vi "Laurel Data GET Top Level.vi"(0 "Laurel IP Address":string="10.0.3.173", 1 "Laurel Serial Commands":T1, 2 "First Call?":bool, 5 "Use Delay":bool, 9 "Serial VISA":refnum<visa-resource-name>, 11 "error in (no error)":errorcluster, 12 "byte count":i32=8, 13 "Laurel Communication Type":string, 14 "All Items Byte Count (Flow Rate)":i32=17) -> (3 "Single Item":dbl, 4 "Flow Rate (Item 1)":dbl, 6 "Gallons (Item 2)":dbl, 8 "Serial VISA Out":refnum<visa-resource-name>, 10 "read buffer":string="0092.3", 15 "error out":errorcluster)   [LabVIEW 2019]
uses:
  Type Definitions/Laurel Serial Commands.ctl
  Type Definitions/Laurel Connection Type.ctl
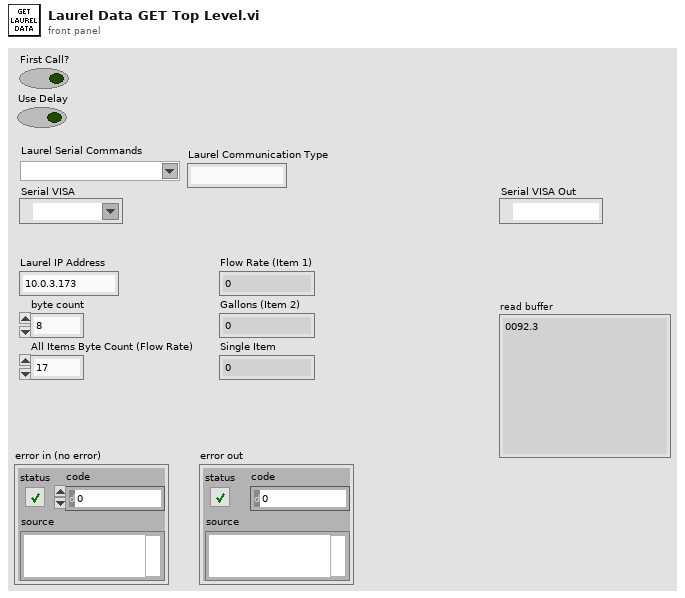
[diagram p1: front panel]
types:
  T1 = typedef "Laurel Serial Commands.ctl" = string
  T2 = typedef "Laurel Connection Type.ctl" = enum16{"Serial", "TCP"}
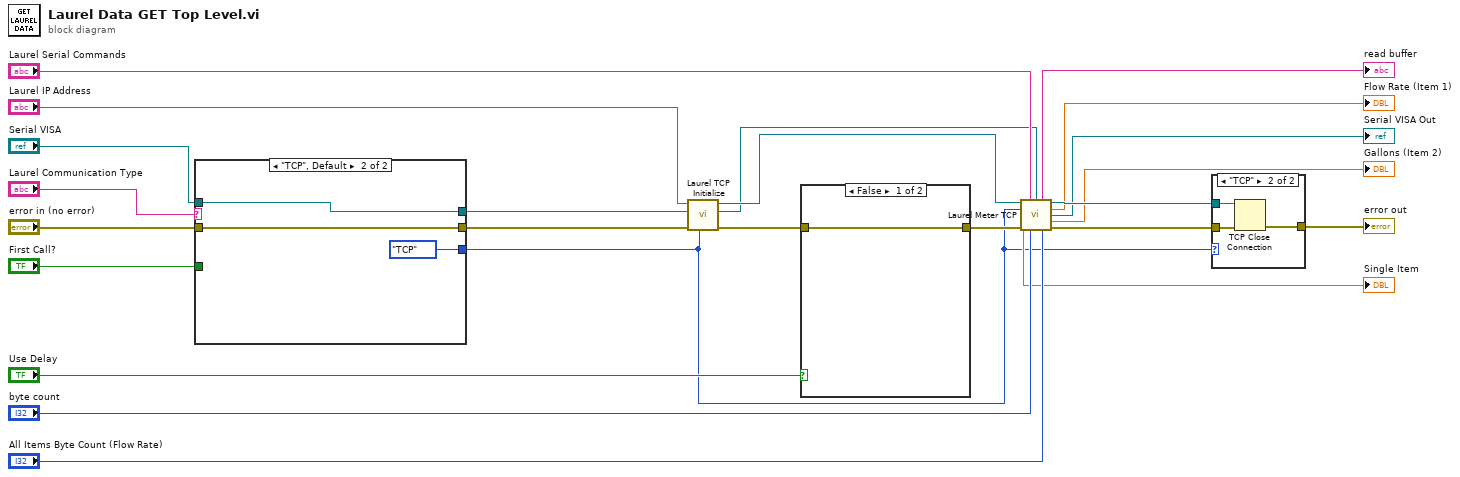
[diagram p0: block diagram]
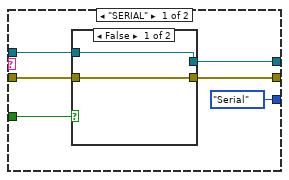
[diagram p2: hidden frame]
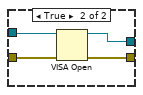
[diagram p3: hidden frame]
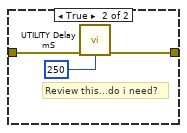
[diagram p5: hidden frame]
diagram:
  n1 = case shown="\"TCP\", Default" "Laurel Communication Type" {
    tunnel: [Laurel_Connection_Type."Serial" ("Connection Type") Laurel_Connection_Type."TCP" ("Connection Type")] -> w1
    tunnel: "error in (no error)" -> [w29 w37]
    tunnel: [w28 w37] -> w5
    tunnel: "Serial VISA" -> [w27 w38]
    tunnel: [w26 w38] -> w2
    tunnel: "First Call?" -> [w25 _]
    frame "SERIAL" {
      n2 = case shown="False" w25 {
        tunnel: [w31 w36] -> w26
        tunnel: w27 -> [w31 w35]
        tunnel: w29 -> [w32 w34]
        tunnel: [w32 w33] -> w28
        frame False {
        }
        frame True {
          n3 = VISA Open(error in (no error)=w34, VISA resource name=w35) -> (VISA resource name=w36:refnum<visa-resource-name>, error out=w33:errorcluster)  [unwired: 3 in]
        }
      }
    }
    frame "TCP", Default {
    }
  }
  n4 = call "Laurel TCP Initialize.vi"("Connection Type"=w1, "Error In"=w5, "Serial VISA"=w2, "Laurel IP Address"="Laurel IP Address") -> ("Error Out"=w12:errorcluster, "Serial VISA Out"=w9:refnum<visa-resource-name>, "Laurel Ref"=w24:refnum<k5>)  [unwired: 5 in]
  n5 = case shown="False" "Use Delay" {
    tunnel: w12 -> [w40 w43]
    tunnel: [w40 w41] -> w11
    frame False {
    }
    frame True {
      # "Review this...do i need?"
      n6 = call "UTILITY Delay mS.vi"("Error In"=w43, "milliseconds to wait"=u32 250) -> ("Error Out"=w41:errorcluster)  [unwired: 13 in]
    }
  }
  n7 = call "Laurel Meter TCP.vi"("TCP Network Connection in"=w24, "Laurel Serial Commands"="Laurel Serial Commands", "Serial VISA"=w9, "Connection Type"=w1, "error in (no error)"=w11, "byte count (Individual)"="byte count", "All Items Byte Count (Flow Rate)"="All Items Byte Count (Flow Rate)") -> ("read buffer"=→"read buffer":string, "TCP Network Connection out"=w23:refnum<k5>, "Flow Rate (Item 1)"=→"Flow Rate (Item 1)":dbl, "Serial VISA Out"=→"Serial VISA Out":refnum<visa-resource-name>, "Single Item"=→"Single Item":dbl, "Gallons (Item 2)"=→"Gallons (Item 2)":dbl, "error out"=w21:errorcluster)  [unwired: 2 in]
  n8 = case shown="\"TCP\"" w1 {
    tunnel: w23 -> [_ w47]
    tunnel: [w44 w46] -> w22
    tunnel: w21 -> [w44 w45]
    frame "Serial", Default {
    }
    frame "TCP" {
      n9 = TCP Close Connection(connection ID=w47, error in (no error)=w45) -> (error out=w46:errorcluster)  [unwired: 1 in, 1 out]
    }
  }
  "error out" <- w22
